vi "Absolute Angle Difference (scalar).vi"(7 "angle units":T1 items=["radian in, radian out", "radian in, degree out", "degree in, degree out", "degree in, radian out"], 10 "angle 2":dbl, 11 "angle 1":dbl) -> (0 "error":i32, 3 "absolute angle difference":dbl)   [LabVIEW 2017, in "NI_AAL_Angle.lvlib"]
doc: "Calculates the absolute difference between two input angles or multiple pairs of input angles.\n\nWire data to any of the angle inputs to determine the polymorphic instance to use or manually select the instance."
uses:
  <vilib>/Analysis/NI_AAL_Angle.lvlib
  <vilib>/Analysis/coordinate.llb/Angle Units.ctl
  <vilib>/Analysis/coordinate.llb/Angle Range (Degree).ctl
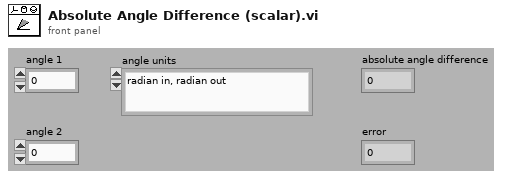
[diagram p1: front panel]
types:
  T1 = typedef "NI_AAL_Angle.lvlib/Angle Units.ctl" = i32
  T2 = typedef "NI_AAL_Angle.lvlib/Angle Range (Degree).ctl" = u16
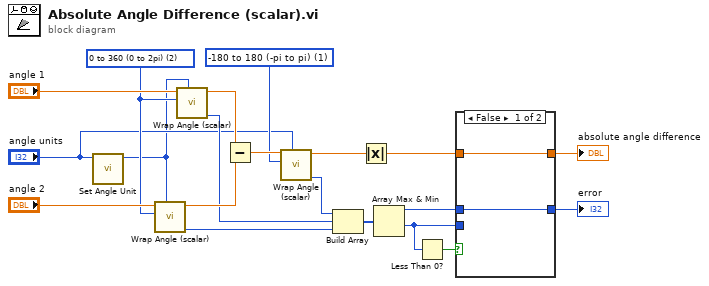
[diagram p0: block diagram]
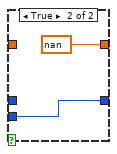
[diagram p2: hidden frame]
diagram:
  w14 = T2 1 items=["none", "-180 to 180 (-pi to pi)", "0 to 360 (0 to 2pi)"] ("angle range")
  w18 = T2 2 items=["none", "-180 to 180 (-pi to pi)", "0 to 360 (0 to 2pi)"] ("angle range")
  n1 = call <vilib>:"Set Angle Unit.vi"("angle units in"="angle units") -> ("angle units out"=w1:T1)  [unwired: 10 in]
  n2 = call <vilib>:"Wrap Angle (scalar).vi"("angle units"=w1, "angle range"=w18, "angle in"="angle 2") -> ("error"=w11:i32, "angle out"=w16:dbl)  [unwired: 7 in]
  n3 = call <vilib>:"Wrap Angle (scalar).vi"("angle units"=w1, "angle range"=w18, "angle in"="angle 1") -> ("error"=w12:i32, "angle out"=w17:dbl)  [unwired: 7 in]
  n4 = Subtract(x=w17, y=w16) -> (x-y=w15:dbl)
  n5 = call <vilib>:"Wrap Angle (scalar).vi"("angle units"="angle units", "angle range"=w14, "angle in"=w15) -> ("error"=w10:i32, "angle out"=w13:dbl)  [unwired: 7 in]
  n6 = Build Array(w10, w12, w11) -> (w9:i32[])
  n7 = Absolute Value(x=w13) -> (abs(x)=w7:dbl)
  n8 = Array Max & Min(array=w9) -> (max value=w3:i32, min value=w5:i32)  [unwired: 2 out]
  n9 = Less Than 0?(x=w5) -> (x < 0?=w8:bool)
  n10 = case shown="False" w8 {
    tunnel: w7 -> [w22 _]
    tunnel: [w22 nan] -> w6
    tunnel: w5 -> [_ w23]
    tunnel: [w21 w23] -> w4
    tunnel: w3 -> [w21 _]
    frame False {
    }
    frame True {
    }
  }
  "absolute angle difference" <- w6
  "error" <- w4
